vi "MANIPULATOR STER PID.vi"(11 "MANIPULATOR wy 3":T1) -> (3 "MANIPULATOR wy 2":T1)   [LabVIEW 2015]
uses:
  <vilib>/addons/control/pid/pid.llb/PID (DBL).vi
  <vilib>/addons/control/pid/NI_PID_pid.lvlib
panel:
  in  "setpoint":dbl format="%.2f"
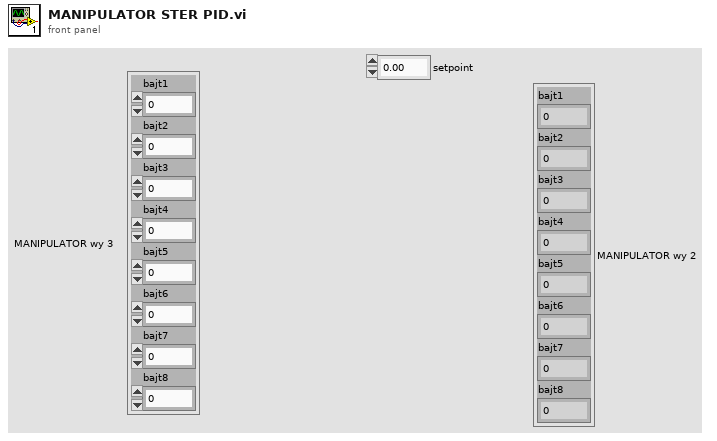
[diagram p1: front panel]
types:
  T1 = cluster{"bajt1":u8, "bajt2":u8, "bajt3":u8, "bajt4":u8, "bajt5":u8, "bajt6":u8, "bajt7":u8, "bajt8":u8}
  T2 = cluster{"bajt1":u8, "bajt2":u8, "bajt3":u8, u8, "bajt5":u8, "bajt6":u8, "bajt7":u8, "bajt8":u8}
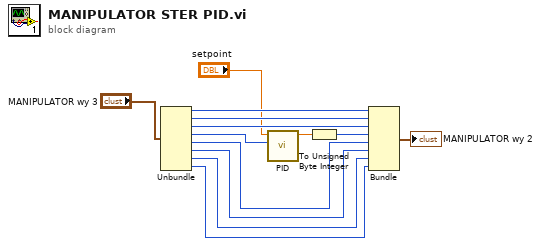
[diagram p0: block diagram]
diagram:
  n1 = Unbundle("MANIPULATOR wy 3") -> ("bajt1"=w11:u8, "bajt2"=w10:u8, "bajt3"=w9:u8, "bajt4"=w2:u8, "bajt5"=w3:u8, "bajt6"=w8:u8, "bajt7"=w7:u8, "bajt8"=w6:u8)
  n2 = call-poly <vilib>:"PID.vi"("process variable"=w2, "setpoint"="setpoint") -> ("output"=w4:dbl)  [unwired: 8 in, 1 out]
  n3 = To Unsigned Byte Integer(number=w4) -> (unsigned 8bit integer=w5:u8)
  n4 = Bundle("bajt1"=w11, "bajt2"=w10, "bajt3"=w9, w5, "bajt5"=w3, "bajt6"=w8, "bajt7"=w7, "bajt8"=w6) -> (→"MANIPULATOR wy 2":T2)  [unwired: 1 in]
